vi "Unwrap position.vi"(11 "all rows":sgl[](array[numeric])) -> (3 "Array":sgl[](array[numeric]))   [LabVIEW 2016]
uses:
  <vilib>/Analysis/NI_AALPro.lvlib
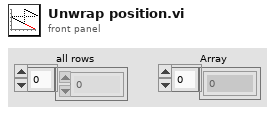
[diagram p1: front panel]
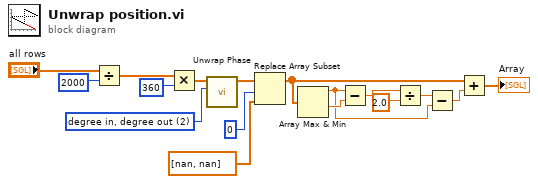
[diagram p0: block diagram]
diagram:
  w12 = 2 items=["radian in, radian out", "radian in, degree out", "degree in, degree out", "degree in, radian out"] ("phase unit")
  n1 = Divide(x="all rows", y=2000) -> (x/y=w16:sgl[])
  n2 = Multiply(x=w16, y=360) -> (x*y=w13:sgl[])
  n3 = call <vilib>:"Unwrap Phase.vi"("phase unit"=w12, "Phase"=w13) -> ("Unwrapped Phase"=w11:dbl[])  [unwired: 8 in, 1 out]
  n4 = Replace Array Subset(array=w11, new element=dbl[] [nan, nan], index=0) -> (w1:dbl[])
  n5 = Array Max & Min(array=w1) -> (max value=w4:dbl, min value=w5:dbl)  [unwired: 2 out]
  n6 = Subtract(x=w4, y=w5) -> (x-y=w8:dbl)
  n7 = Divide(x=w8, y=2.0) -> (x/y=w2:dbl)
  n8 = Subtract(x=w2, y=w4) -> (x-y=w3:dbl)
  n9 = Add(x=w1, y=w3) -> (x+y=→"Array":dbl[])
